vi "Log DSF Paths.vi"(8 "error in (no error)":errorcluster, 11 "Item Ref in":T1 format="%.0x") -> (0 "error out":errorcluster, 3 "Item Ref out":T1 format="%.0x")   [LabVIEW 2017, in "DSF Engine.lvlib"]
uses:
  DSF Engine.lvlib
  <vilib>/NI Veristand/Custom Device API/Custom Device Item Ref.ctl
  Shared/DSF Shared.lvlib
  <vilib>/NI Veristand/Custom Device API/Custom Device API.lvlib
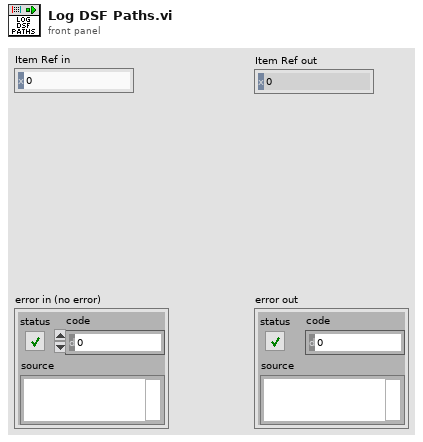
[diagram p1: front panel]
types:
  T1 = typedef "Custom Device API.lvlib/Custom Device Item Ref.ctl" = u64
  T2 = enum16{"open", "replace", "create", "open or create", "replace or create", "replace or create with confirmation"}
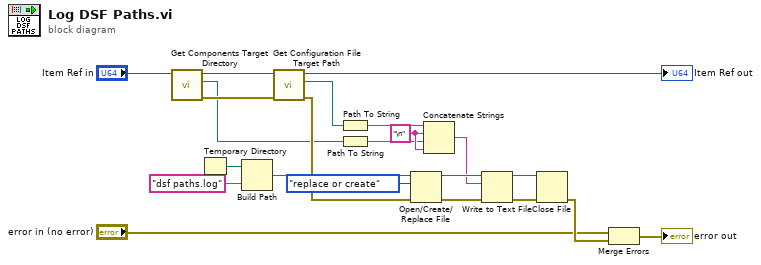
[diagram p0: block diagram]
diagram:
  w13 = "\n" ("string")
  n1 = call "Get Components Target Directory.vi"("Item Ref in"="Item Ref in") -> ("error out"=w6:errorcluster, "components target directory"=w4:path, "Item Ref out"=w7:T1)  [unwired: 8 in]
  n2 = Temporary Directory() -> (w10:path)
  n3 = Build Path(base path=w10, name or relative path="dsf paths.log" ("file path (use dialog)")) -> (appended path=w8:path)
  n4 = call "Get Configuration File Target Path.vi"("error in (no error)"=w6, "Item Ref in"=w7) -> ("error out"=w22:errorcluster, "configuration target path"=w5:path, "Item Ref out"=→"Item Ref out":T1)  [unwired: 7 in]
  n5 = Path To String(path=w5) -> (string=w14:string)
  n6 = Path To String(path=w4) -> (string=w12:string)
  n7 = Open/Create/Replace File(file path (use dialog)=w8, error in=w22, operation (0:open)=T2."replace or create") -> (refnum out=w17:refnum<file>, error out=w18:errorcluster)  [unwired: 3 in, 1 out]
  n8 = Concatenate Strings(w14, w13, w12, w13) -> (w11:string)
  n9 = Write to Text File(file (use dialog)=w17, text=w11, error in=w18) -> (refnum out=w15:refnum<file>, error out=w16:errorcluster)  [unwired: 1 in, 1 out]
  n10 = Close File(refnum=w15, error in=w16) -> (error out=w3:errorcluster)  [unwired: 1 out]
  n11 = Merge Errors("error in (no error)", w3) -> (→"error out":errorcluster)
